vi "Builder Status.Create.vi"(8 "error in (no error)":errorcluster, 10 "Build Durations Pointer":refnum<class "Memory.Pointer.U32.lvclass">, 11 "Builder Status type":refnum<class "Builder Status.lvclass">) -> (0 "error out":errorcluster, 3 "Builder Status":refnum<class "Builder Status.lvclass">)   [LabVIEW 2016, in "DSF.Engine.lvlib" / "Builder Status.lvclass"]
uses:
  Builder Status.lvclass
  Submodules/Memory/Source/Classes/Standard Types/Memory.Pointer.U32.lvclass
  Builder Status.lvclass/Builder Status.ctl
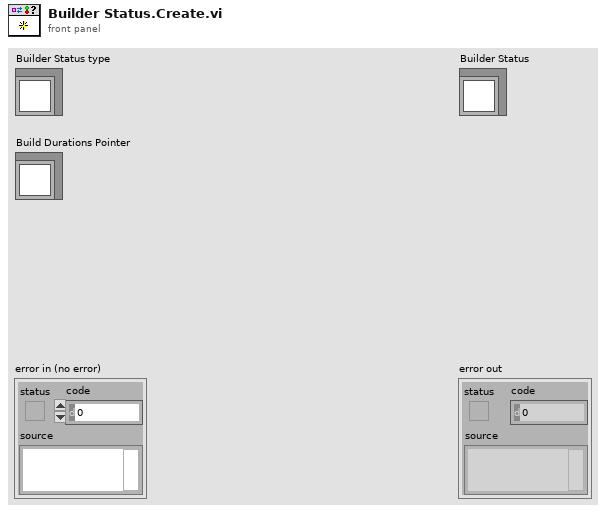
[diagram p1: front panel]
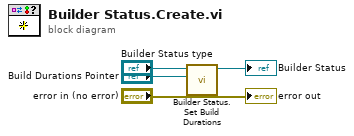
[diagram p0: block diagram]
diagram:
  n1 = call "Builder Status.Set Build Durations.vi"("Build Durations"="Build Durations Pointer", "Builder Status in"="Builder Status type") -> ("Builder Status out"=→"Builder Status":refnum<class "Builder Status.lvclass">)  [unwired: 9 in]
  "error out" <- "error in (no error)"
